vi "update_status.vi"(8 "error in (no error)":errorcluster, 10 "status":string, 11 "events":T1) -> (0 "error out":errorcluster, 3 "events_out":T1)   [LabVIEW 2018]
uses:
  swabian_events_tdef.ctl
  update_chart_tdef.ctl
  channel_data_tdef.ctl
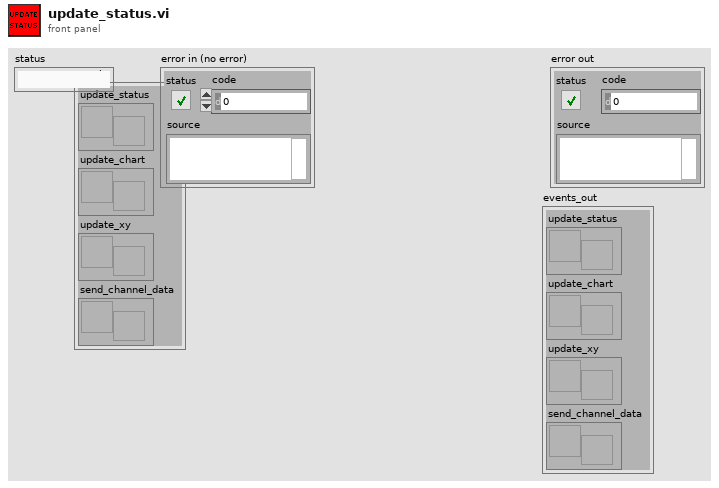
[diagram p1: front panel]
types:
  T1 = typedef "swabian_events_tdef.ctl" = cluster{"update_status":refnum<user-event>, "update_chart":refnum<user-event>, "update_xy":refnum<user-event>, "send_channel_data":refnum<user-event>}
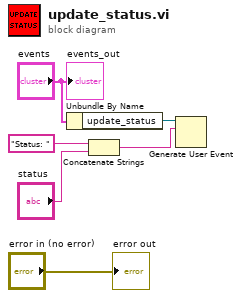
[diagram p0: block diagram]
diagram:
  n1 = Unbundle By Name("events") -> ("update_status"=w5:refnum<user-event>)
  n2 = Concatenate Strings("Status: " ("string"), "status") -> (w2:string)
  n3 = Generate User Event(user event=w5, event data cluster=w2) -> ()  [unwired: 2 in, 2 out]
  "error out" <- "error in (no error)"
  "events_out" <- "events"
